vi "Intake Mode Selector.vi"(8 "Semi Auto?":bool, 9 "Manual?":bool) -> (2 "Intake Mode":T1)   [LabVIEW 2017]
uses:
  Common Code/Intake Mode.ctl
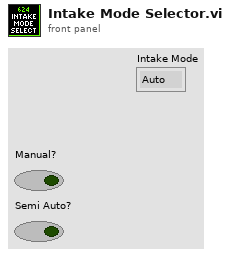
[diagram p1: front panel]
types:
  T1 = typedef "Intake Mode.ctl" = enum16{"Auto", "Semi Auto", "Manual"}
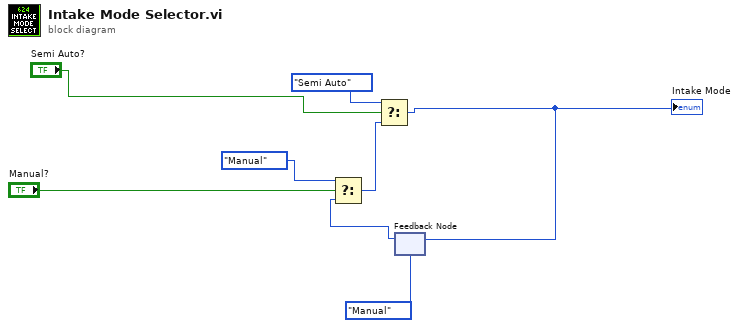
[diagram p0: block diagram]
diagram:
  n1 = feedback #1(Intake_Mode."Manual" ("Intake Mode")) -> (w3:T1)
  n2 = Select(t=Intake_Mode."Manual" ("Intake Mode"), s="Manual?", f=w3) -> (s? t:f=w6:T1)
  n3 = Select(t=Intake_Mode."Semi Auto" ("Intake Mode"), s="Semi Auto?", f=w6) -> (s? t:f=w1:T1)
  "Intake Mode" <- w1
  n4 = feedback-in #1(w1) -> ()
